vi "PropertyTypeToString.vi"(4 "Property Type":T1 items=["Bool"=0, "Int"=1, "Float"=2, "String"=3, "List"=4, "Dict"=5, "Ratio"=6, "Procedure"=7, "Object"=8, "Function"=10, "Struct"=12, "Enumeration"=13, "Reference"=4096, "IndexSelection"=4097, "TypeSelection"=4098, "SparseSelection"=4099, "Undefined"=65535]) -> (1 "String":string)   [LabVIEW 2022 SP3, in "Property Editor.lvlib"]
uses:
  <instrlib>/openDAQ/Examples/Property Editor/Property Editor.lvlib
  <instrlib>/openDAQ/Public/TypeDef/PropertyType.ctl
  <instrlib>/openDAQ/openDAQ.lvlib
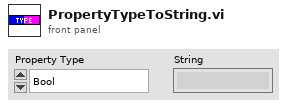
[diagram p1: front panel]
types:
  T1 = typedef "openDAQ.lvlib/PropertyType.ctl" = u16
  T2 = typedef "LVStringsAndValuesArrayTypeDef_U16.ctl" = cluster{"String":string, "Value":u16}[]
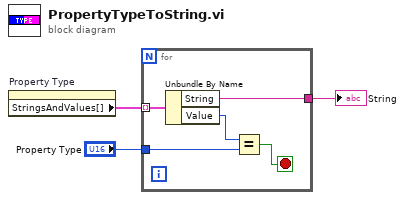
[diagram p0: block diagram]
diagram:
  n1 = property on="Property Type" class="Ring (strict)"() -> ("StringsAndValues[]"=w3:T2)  [unwired: 2 in, 2 out]
  n2 = for {
    tunnel: w3 -> [w8] mode=indexing
    tunnel: [w7] -> w2
    tunnel: "Property Type" -> [w5]
    stop <- w4 stop-if-true
    n3 = Unbundle By Name(w8) -> ("String"=w7:string, "Value"=w6:u16)
    n4 = Equal?(x=w6, y=w5) -> (x = y?=w4:bool)
  }
  "String" <- w2
